vi "Auton Data.vi"(8 "power":dbl[](array[numeric]), 9 "time/distance":dbl[](array[numeric]), 10 "Heading":dbl[](array[numeric]), 11 "primitive ID":i16[](array[numeric])) -> ()   [LabVIEW 2012]
uses:
  <vilib>/Rock Robotics/WPI/DriverStation/DriverStationLCD/WPI_DriverStationLCDLCDLine.ctl
  Begin/Global Variables.vi
panel:
  out "Heading":dbl
  out "Distance/Time":dbl
  out "Power":dbl
  out "ArrayIndex":u16
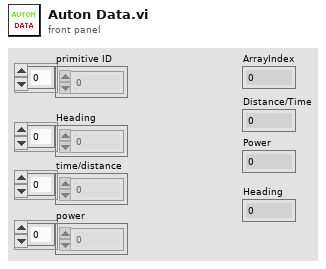
[diagram p1: front panel]
types:
  T1 = typedef "WPI_DriverStationLCDLCDLine.ctl" = enum16{"Main - Line 1", "User - Line 2", "User - Line 3", "User - Line 4", "User - Line 5", "User - Line 6"}
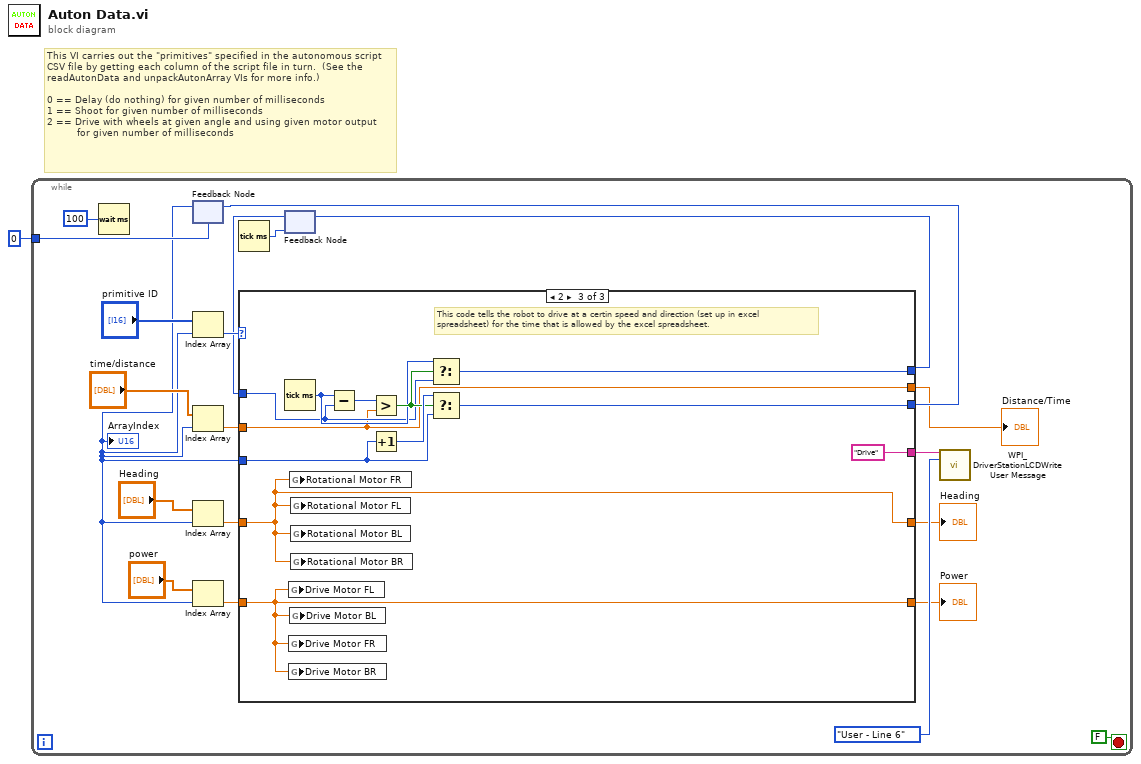
[diagram p0: block diagram]
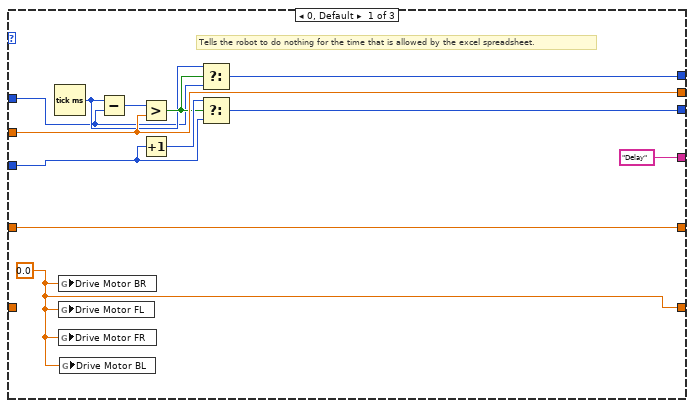
[diagram p2: hidden frame]
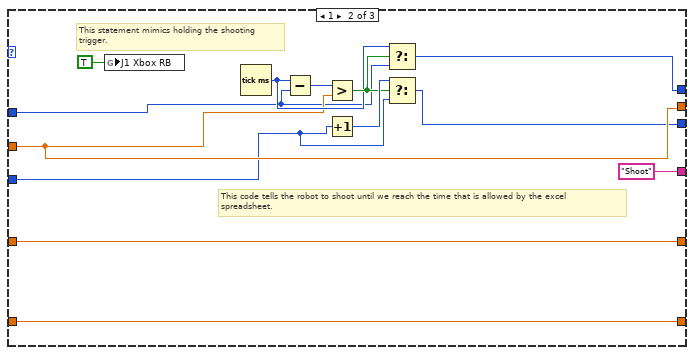
[diagram p3: hidden frame]
diagram:
  # "This VI carries out the \"primitives\" specified in the autonomous script CSV file by getting each column of the script file in turn.  (See the\nreadAutonData and unpackAutonArray VIs for more info.)\n\n0 == Delay (do nothing) for given number of milliseconds\n1 == Shoot for given number of milliseconds\n2 == Drive with wheels at given angle and using given motor output\n          for given number of milliseconds"
  n1 = while {
    tunnel: 0 -> [w15]
    stop <- FALSE stop-if-true
    n2 = Wait (ms)(milliseconds to wait=u32 100) -> ()  [unwired: 1 out]
    n3 = feedback #1(w15) -> (w5:i32)
    "ArrayIndex" <- w5
    n4 = Index Array(array="primitive ID", index=w5) -> (element=w6:i16)
    n5 = Index Array(array="time/distance", index=w5) -> (element=w9:dbl)
    n6 = Index Array(array="Heading", index=w5) -> (element=w7:dbl)
    n7 = Index Array(array="power", index=w5) -> (element=w11:dbl)
    n8 = Tick Count (ms)() -> (millisecond timer value=w4:u32)
    n9 = feedback #2(w4) -> (w3:u32)
    n10 = case shown="2" w6 {
      tunnel: ["Delay" ("line text") "Shoot" ("line text") "Drive" ("line text")] -> w14
      tunnel: [w31 w35 w48] -> w13
      tunnel: [w24 w46 w57] -> w12
      tunnel: w11 -> [_ w46 w57]
      tunnel: [w32 w39 w50] -> w10
      tunnel: w9 -> [w32 w39 w50]
      tunnel: [w23 w45 w58] -> w8
      tunnel: w7 -> [w23 w45 w58]
      tunnel: w5 -> [w29 w38 w49]
      tunnel: w3 -> [w26 w37 w52]
      tunnel: [w25 w36 w51] -> w2
      frame 0, Default {
        w24 = 0.0
        # "Tells the robot to do nothing for the time that is allowed by the excel spreadsheet."
        n11 = Tick Count (ms)() -> (millisecond timer value=w27:u32)
        n12 = global write "Global Variables.vi" "Drive Motor BR"(w24) -> ()
        n13 = global write "Global Variables.vi" "Drive Motor FL"(w24) -> ()
        n14 = global write "Global Variables.vi" "Drive Motor FR"(w24) -> ()
        n15 = global write "Global Variables.vi" "Drive Motor BL"(w24) -> ()
        n16 = Subtract(x=w27, y=w26) -> (x-y=w33:u32)
        n17 = Greater?(x=w33, y=w32) -> (0:w28:bool)
        n18 = Increment(x=w29) -> (x+1=w30:i32)
        n19 = Select(t=w27, s=w28, f=w26) -> (s? t:f=w25:u32)
        n20 = Select(t=w30, s=w28, f=w29) -> (s? t:f=w31:i32)
      }
      frame 1 {
        # "This statement mimics holding the shooting\ntrigger."
        # "This code tells the robot to shoot until we reach the time that is allowed by the excel\nspreadsheet."
        n21 = global write "Global Variables.vi" "J1 Xbox RB"(TRUE ("Shoot trigger")) -> ()
        n22 = Tick Count (ms)() -> (millisecond timer value=w40:u32)
        n23 = Subtract(x=w40, y=w37) -> (x-y=w43:u32)
        n24 = Greater?(x=w43, y=w39) -> (0:w41:bool)
        n25 = Increment(x=w38) -> (x+1=w42:i32)
        n26 = Select(t=w40, s=w41, f=w37) -> (s? t:f=w36:u32)
        n27 = Select(t=w42, s=w41, f=w38) -> (s? t:f=w35:i32)
      }
      frame 2 {
        # "This code tells the robot to drive at a certin speed and direction (set up in excel\nspreadsheet) for the time that is allowed by the excel spreadsheet."
        n28 = Tick Count (ms)() -> (millisecond timer value=w53:u32)
        n29 = global write "Global Variables.vi" "Drive Motor FL"(w57) -> ()
        n30 = global write "Global Variables.vi" "Drive Motor FR"(w57) -> ()
        n31 = global write "Global Variables.vi" "Drive Motor BR"(w57) -> ()
        n32 = global write "Global Variables.vi" "Rotational Motor FR"(w58) -> ()
        n33 = global write "Global Variables.vi" "Drive Motor BL"(w57) -> ()
        n34 = global write "Global Variables.vi" "Rotational Motor FL"(w58) -> ()
        n35 = global write "Global Variables.vi" "Rotational Motor BL"(w58) -> ()
        n36 = global write "Global Variables.vi" "Rotational Motor BR"(w58) -> ()
        n37 = Subtract(x=w53, y=w52) -> (x-y=w56:u32)
        n38 = Greater?(x=w56, y=w50) -> (0:w54:bool)
        n39 = Increment(x=w49) -> (x+1=w55:i32)
        n40 = Select(t=w53, s=w54, f=w52) -> (s? t:f=w51:u32)
        n41 = Select(t=w55, s=w54, f=w49) -> (s? t:f=w48:i32)
      }
    }
    "Heading" <- w8
    "Distance/Time" <- w10
    "Power" <- w12
    n42 = feedback-in #1(w13) -> ()
    n43 = feedback-in #2(w2) -> ()
    n44 = call <vilib>:"WPI_DriverStationLCDWrite User Message.vi"("line text"=w14, "line"=WPI_DriverStationLCDLCDLine."User - Line 6") -> ()  [unwired: 13 in, 1 out]
  }
